vi "only_wheel_turn.vi"() -> ()   [LabVIEW 2019]
uses:
  <vilib>/Platform/TimedLoop/XDataNode/timing_clust.ctl
  <vilib>/Platform/TimedLoop/XDataNode/nitl_modes.ctl
  <vilib>/Platform/TimedLoop/XDataNode/wakeup.ctl
  <vilib>/FPGAPlugInAG/myRIO-1900/niLvFpga_Open_myRIO-1900.vi
  <vilib>/rvi/interface/common/dynamic/niFpgaDynamicAddResources.vi
  <vilib>/Utility/error.llb/Error Cluster From Error Code.vi
  <vilib>/rvi/errors/niLvFpgaAdjustHostInterfaceError.vi
  <vilib>/FPGAPlugInAG/Dynamic/niLvFpga_Close_Dynamic.vi
  <vilib>/Platform/TimedLoop/XDataNode/XDataNode.xnode
  <vilib>/rvi/interface/nirviOpenFPGA/nirviOpenFPGA.xnode
  FPGA Bitfiles/capstone_FPGATarget_encoderFPGA_AeXAVEDpCcY.lvbitx
  encoder_FPGA.vi
  <vilib>/rvi/interface/nirviReadWriteControl/nirviReadWriteControl.xnode
  <vilib>/rvi/interface/nirviCloseFPGA/nirviCloseFPGA.xnode
  <vilib>/Platform/TimedLoop/XDataNode/XDNodeRunTimeDep.lvlib
  <vilib>/rvi/interface/Simulation/niFpgaSimulationCallBeginRW.vi
  NiFpgaLv.dll
panel:
  in  "신중하게 눌러야하는 버튼 ㄹㅇ":bool
  out "i count":i32=73647
  out "불리언 2":bool
  out "불리언":bool=TRUE
  out "둘 다 돌았나?":bool=TRUE
  in  "정지":bool
  in  "wanted angle(deg)":dbl=45.0
  in  "wanted angle":dbl[](array[numeric])
  out "mm/ms":dbl
  out "R_이동 거리":dbl=-191.70651751873433
  out "R_Encoder":i32
  out "L_이동 거리":dbl=-244.45797535945857
  out "L_encoder":i32
  out "타임아웃":i32=-1
  out "x > y?":bool
  # "pwm\n3000"
  # "mm/ms\n0.25"
  # "F일 때 앞으로 돌고, T일 때 뒤로 돎"
  # "k"
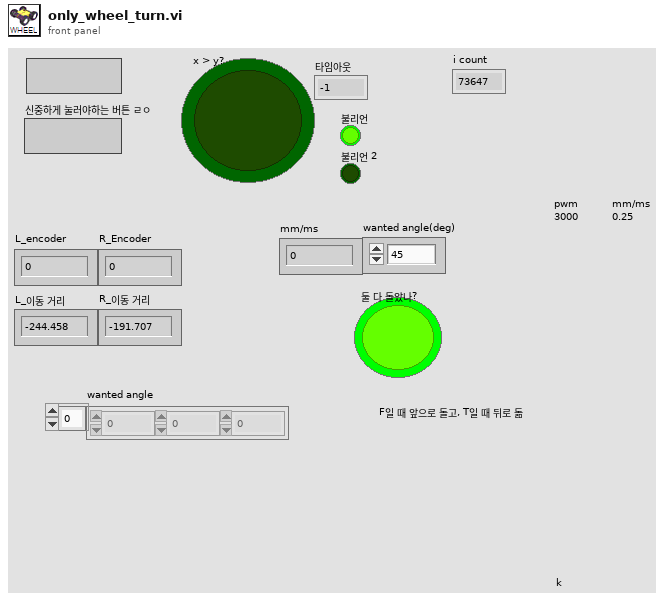
[diagram p1: front panel]
types:
  T1 = typedef "XDNodeRunTimeDep.lvlib/timing_clust.ctl" = cluster{"Expected End [f-1]":u64, "Actual End [f-1]":u64, "Finished Late? [f-1]":bool, "Expected End [i-1]":u64, "Actual End [i-1]":u64, "Finished Late? [i-1]":bool, "Expected Start [i]":u64, "Actual Start [i]":u64, "Expected Start [f]":u64, "Actual Start [f]":u64, "Source Name":string, "Structure Name":string, "Period":i64, "Deadline":i64, "Offset":i64, "Start":i64, "Priority":i32, "Timeout":i32, "Mode":T2, "Wakeup Reason":T3, "Error":errorcluster, "Source Type":string, "Secondary Source Type":string, "Global End Time":u64, "Global Start Time":u64, "Frame Duration":u64, "Iteration Duration":u64, "Assigned CPU":i32, "I/O Scan Engine Mode":u32}
  T2 = typedef "XDNodeRunTimeDep.lvlib/nitl_modes.ctl" = enum32{"No Change", "Process missed periods, maintain original phase", "Discard missed periods, maintain original phase", "Process missed periods, ignore original phase", "Discard missed periods, ignore original phase"}
  T3 = typedef "XDNodeRunTimeDep.lvlib/wakeup.ctl" = enum32{"Normal", "Aborted", "Asynchronous wakeup", "Timing source error", "Timed loop error", "Timeout"}
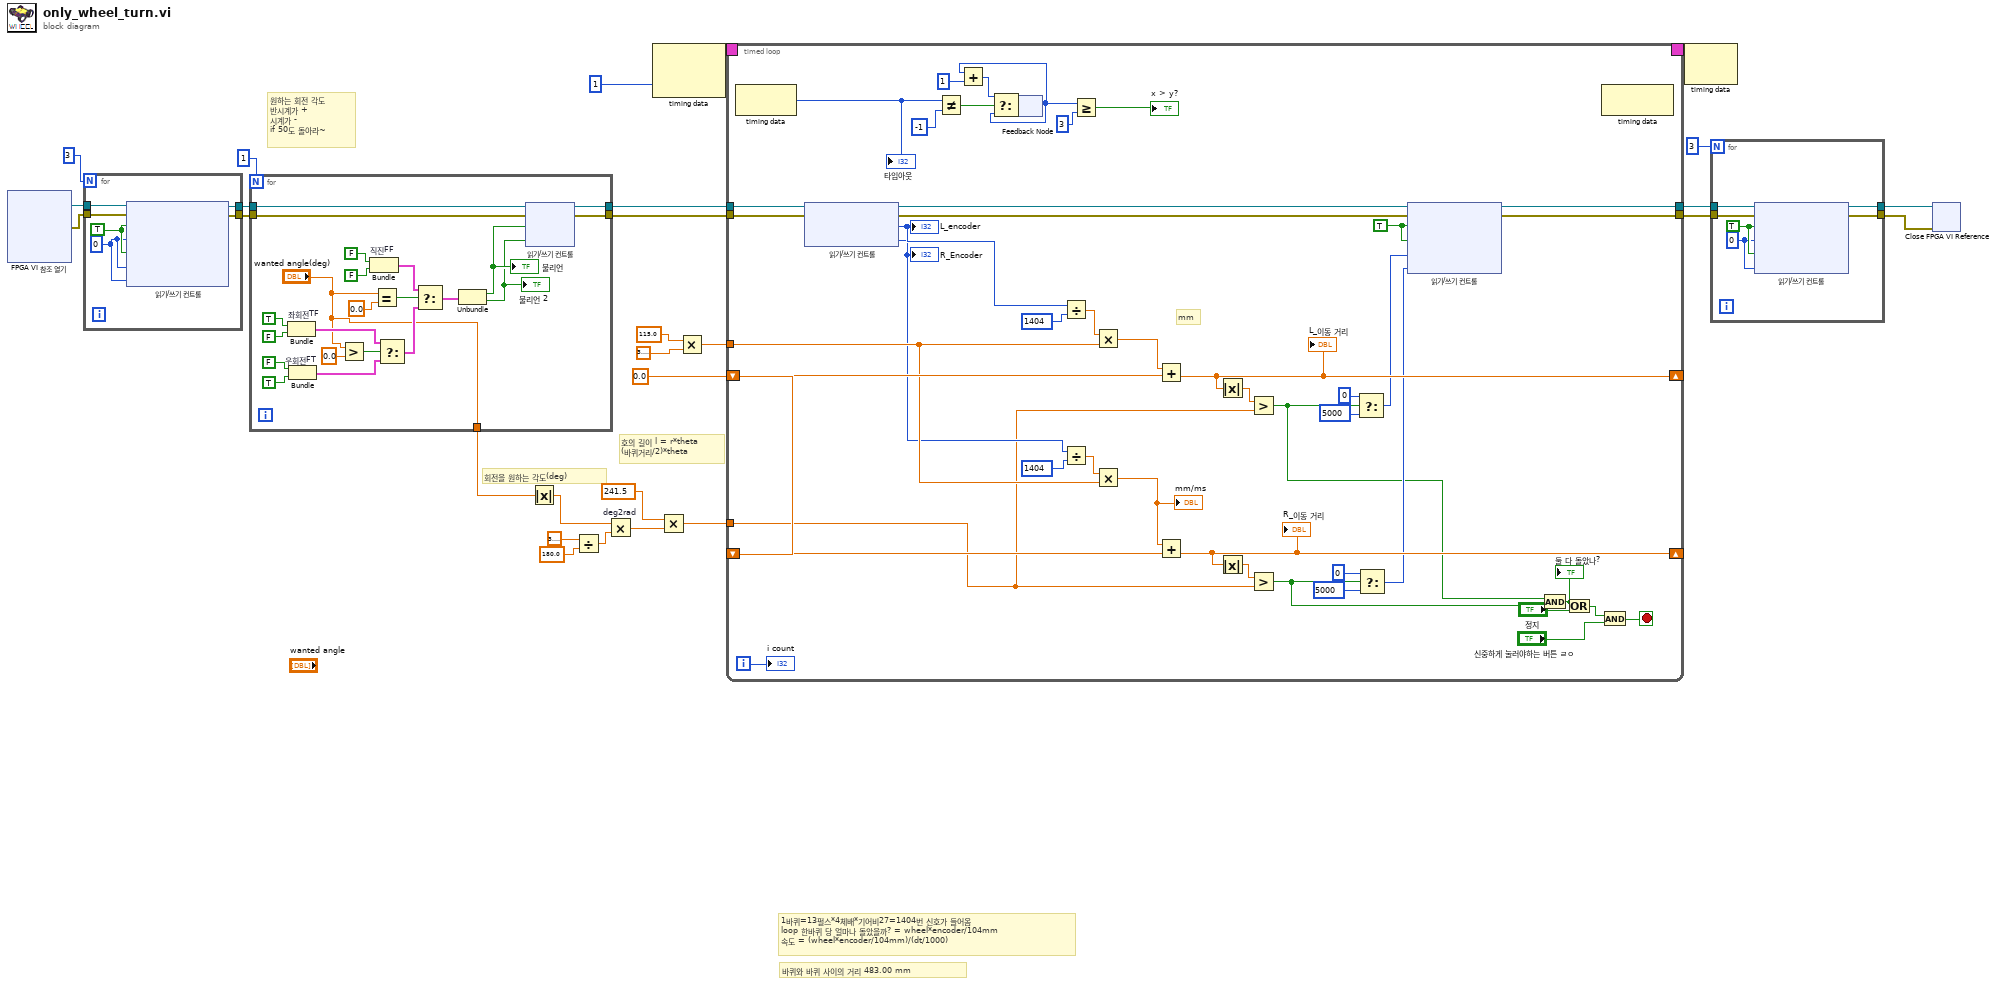
[diagram p0: block diagram]
diagram:
  w19 = 0.0
  # "원하는 회전 각도\n반시계가 +\n시계가 -\nif 50도 돌아라~"
  # "호의 길이 l = r*theta\n(바퀴거리/2)*theta"
  # "회전을 원하는 각도(deg)"
  # "바퀴와 바퀴 사이의 거리 483.00 mm"
  # "1바퀴=13펄스*4체배*기어비27=1404번 신호가 들어옴\nloop 한바퀴 당 얼마나 돌았을까? = wheel*encoder/104mm\n속도 = (wheel*encoder/104mm)/(dt/1000)"
  n1 = xnode "FPGA VI 참조 열기"() -> ("FPGA VI 참조 출력"=w18:refnum<k20>, "에러 출력"=w17:errorcluster)  [unwired: 2 in]
  n2 = for {
    N: 3 -> [_]
    tunnel: [w34] -> w12
    tunnel: [w33] -> w11
    tunnel: w18 -> [w30]
    tunnel: w17 -> [w29]
    w31 = 0 ("pwm input(escon)")
    w32 = TRUE ("encoder reset")
    n3 = xnode "읽기/쓰기 컨트롤"("FPGA VI 참조 입력"=w30, "에러 입력"=w29, "encoder reset"=w32, "pwm input"=w31, "R_encoder reset"=w32, "R_pwm input"=w31, "직동_pwm input"=w31) -> ("FPGA VI 참조 출력"=w34:refnum<k20>, "에러 출력"=w33:errorcluster)
  }
  n4 = for {
    N: 1 -> [_]
    tunnel: [w39] -> w14
    tunnel: [w38] -> w13
    tunnel: w12 -> [w37]
    tunnel: w11 -> [w36]
    tunnel: ["wanted angle(deg)"] -> w1
    n5 = Bundle "좌회전TF"(TRUE, FALSE) -> (w42:cluster{bool, bool})  [unwired: 1 in]
    n6 = Bundle "우회전FT"(FALSE, TRUE) -> (w41:cluster{bool, bool})  [unwired: 1 in]
    n7 = Greater?(x="wanted angle(deg)", y=0.0) -> (0:w44:bool)
    n8 = Bundle "직진FF"(FALSE, FALSE) -> (w48:cluster{bool, bool})  [unwired: 1 in]
    n9 = Equal?(x="wanted angle(deg)", y=0.0) -> (x = y?=w56:bool)
    n10 = Select(t=w42, s=w44, f=w41) -> (s? t:f=w40:cluster{bool, bool})
    n11 = Select(t=w48, s=w56, f=w40) -> (s? t:f=w47:cluster{bool, bool})
    n12 = Unbundle(w47) -> (w46:bool, w45:bool)
    "불리언" <- w46
    "불리언 2" <- w45
    n13 = xnode "읽기/쓰기 컨트롤"("FPGA VI 참조 입력"=w37, "에러 입력"=w36, "L_dir"=w46, "R_dir"=w45) -> ("FPGA VI 참조 출력"=w39:refnum<k20>, "에러 출력"=w38:errorcluster)
  }
  n14 = Absolute Value(x=w1) -> (abs(x)=w2:dbl)
  n15 = Divide(x=3.141592653589793, y=180.0) -> (x/y=w7:dbl)
  n16 = Multiply "deg2rad"(x=w2, y=w7) -> (x*y=w5:dbl)
  n17 = node-c288(i64 1 ("주기")) -> (w28:T1)  [unwired: 1 in]
  n18 = Multiply(x=241.5, y=w5) -> (x*y=w4:dbl)
  n19 = Multiply(x=115.0, y=3.141592653589793) -> (x*y=w21:dbl)
  n20 = timed-loop {
    timing: w28 -> [_]
    timing-out: [_] -> w27
    tunnel: [w93] -> w26
    tunnel: [w92] -> w25
    tunnel: w21 -> [w86]
    shift-right: [w90] -> _
    shift-left: w19 -> [w87]
    shift-right: [w89] -> _
    shift-left: w19 -> [w88]
    tunnel: w14 -> [w83]
    tunnel: w13 -> [w82]
    tunnel: w4 -> [w81]
    i -> [w58]
    stop <- w62 stop-if-true
    w91 = TRUE ("encoder reset")
    # "mm"
    n21 = node-c288() -> (w102:i32)  [unwired: 1 in]
    "타임아웃" <- w102
    n22 = xnode "읽기/쓰기 컨트롤"("FPGA VI 참조 입력"=w83, "에러 입력"=w82) -> ("FPGA VI 참조 출력"=w60:refnum<k20>, "에러 출력"=w59:errorcluster, "Encoder  (4x)"=w85:i32, "R_Encoder  (4x)"=w84:i32)
    "L_encoder" <- w85
    "R_Encoder" <- w84
    n23 = Not Equal?(x=w102, y=-1) -> (x != y?=w100:bool)
    n24 = feedback #1() -> (w96:u8)  [unwired: 1 in]
    n25 = Add(x=w96, y=u8 1) -> (x+y=w99:u8)
    n26 = Select(t=w99, s=w100, f=w96) -> (s? t:f=w98:u8)
    n27 = feedback-in #1(w98) -> ()
    n28 = Divide(x=w85, y=1404) -> (x/y=w79:dbl)
    n29 = Divide(x=w84, y=1404) -> (x/y=w75:dbl)
    n30 = Greater Or Equal?(x=w96, y=u8 3) -> (x >= y?=→"x > y?":bool)
    n31 = Multiply(x=w79, y=w86) -> (x*y=w73:dbl)
    n32 = Multiply(x=w75, y=w86) -> (x*y=w76:dbl)
    "mm/ms" <- w76
    n33 = Add(x=w73, y=w87) -> (x+y=w90:dbl)
    "L_이동 거리" <- w90
    n34 = Add(x=w76, y=w88) -> (x+y=w89:dbl)
    "R_이동 거리" <- w89
    n35 = Absolute Value(x=w90) -> (abs(x)=w78:dbl)
    n36 = Absolute Value(x=w89) -> (abs(x)=w74:dbl)
    n37 = Greater?(x=w78, y=w81) -> (0:w65:bool)
    n38 = Greater?(x=w74, y=w81) -> (0:w66:bool)
    n39 = Select(t=0, s=w65, f=5000) -> (s? t:f=w67:i32)
    n40 = Select(t=0, s=w66, f=5000) -> (s? t:f=w70:i32)
    n41 = xnode "읽기/쓰기 컨트롤"("FPGA VI 참조 입력"=w60, "에러 입력"=w59, "encoder reset"=w91, "R_encoder reset"=w91, "pwm input"=w67, "R_pwm input"=w70) -> ("FPGA VI 참조 출력"=w93:refnum<k20>, "에러 출력"=w92:errorcluster)
    n42 = And(x=w65, y=w66) -> (x .and. y?=w64:bool)
    "둘 다 돌았나?" <- w64
    n43 = Or(x=w64, y="정지") -> (x .or. y?=w61:bool)
    n44 = And(x=w61, y="신중하게 눌러야하는 버튼 ㄹㅇ") -> (x .and. y?=w62:bool)
    n45 = node-c288() -> ()  [unwired: 1 in, 1 out]
    "i count" <- w58
  }
  n46 = node-c288(w27) -> ()  [unwired: 1 out]
  n47 = for {
    N: 3 -> [_]
    tunnel: w26 -> [w111]
    tunnel: w25 -> [w110]
    tunnel: [w107] -> w16
    tunnel: [w106] -> w15
    w108 = 0 ("pwm input(escon)")
    w109 = TRUE ("encoder reset")
    n48 = xnode "읽기/쓰기 컨트롤"("FPGA VI 참조 입력"=w111, "에러 입력"=w110, "encoder reset"=w109, "pwm input"=w108, "R_encoder reset"=w109, "R_pwm input"=w108) -> ("FPGA VI 참조 출력"=w107:refnum<k20>, "에러 출력"=w106:errorcluster)
  }
  n49 = xnode "Close FPGA VI Reference"("FPGA VI 참조 입력"=w16, "에러 입력"=w15) -> ()  [unwired: 1 out]
